vi "measurement.vi"(6 "error in (no error)":errorcluster, 9 "Experiment.lvclass":refnum<class "Experiment.lvclass">) -> (0 "error out":errorcluster, 3 "Experiment out":refnum<class "Experiment.lvclass">)   [LabVIEW 2013, in "Experiment.lvclass"]
doc: "I Description:\nThis example uses a script to manage the generation of a dynamic pattern at a specified clock rate.\n\nII Instructions for Running:\n1. Enter the digital channels on the hardware device to generate digital pattern in the Channel List control.\n2. Specify the clock rate for the generation in the Clock Rate control.\n3. Click the Stop button when you want to stop the generation\n\nIII Block Diagram Steps:\n1. Initialize for a generation session.\n2. Assign specified channels in Channel List for dynamic operation.\n3. Configure the Sample clock to use the onboard clock, and configure the clock rate.\n4. Set the generation mode to Scripted.\n5. Query the Data Width property to determine which Write function to use.\nNote: Different devices have different default values for the Data Width property. If you know the Data Width of your device, you may omit the property node and case structure.\n6. Write digital patterns to the onboard memory of the digital device.\n7. Write the script to the onboard memory.\n8. Initiate dynamic pattern generation.\n9. Wait until the Stop button is clicked or an error occurs, and exit the While loop. \n The niHSDIO Is Done VI is used in the while loop to check only for errors.\n10. Abort generation and close the session.\n\nIV I/O Connections Overview:\nMake connections from output terminals to match the channels specified by Channel List. In this example, the digital pattern is generated from the first 16 digital channels of the device."
uses:
  Experiment.lvclass
  <vilib>/Platform/TimedLoop/XDataNode/timing_clust.ctl
  <vilib>/Platform/TimedLoop/XDataNode/nitl_modes.ctl
  <vilib>/Platform/TimedLoop/XDataNode/wakeup.ctl
  Globals.vi
  <vilib>/platform/TimedLoop/XDataNode/XDataNode.xnode
  <vilib>/Platform/TimedLoop/XDataNode/XDNodeRunTimeDep.lvlib
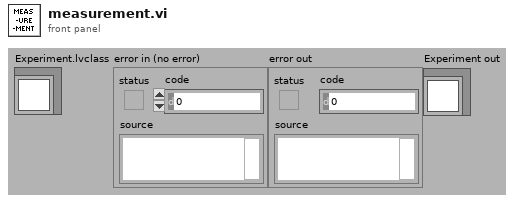
[diagram p1: front panel]
types:
  T1 = typedef "XDNodeRunTimeDep.lvlib/timing_clust.ctl" = cluster{"Expected End [f-1]":u64, "Actual End [f-1]":u64, "Finished Late? [f-1]":bool, "Expected End [i-1]":u64, "Actual End [i-1]":u64, "Finished Late? [i-1]":bool, "Expected Start [i]":u64, "Actual Start [i]":u64, "Expected Start [f]":u64, "Actual Start [f]":u64, "Source Name":string, "Structure Name":string, "Period":i64, "Deadline":i64, "Offset":i64, "Start":i64, "Priority":i32, "Timeout":i32, "Mode":T2, "Wakeup Reason":T3, "Error":errorcluster, "Source Type":string, "Secondary Source Type":string, "Global End Time":u64, "Global Start Time":u64, "Frame Duration":u64, "Iteration Duration":u64, "Assigned CPU":i32, "I/O Scan Engine Mode":u32}
  T2 = typedef "XDNodeRunTimeDep.lvlib/nitl_modes.ctl" = enum32{"No Change", "Process missed periods, maintain original phase", "Discard missed periods, maintain original phase", "Process missed periods, ignore original phase", "Discard missed periods, ignore original phase"}
  T3 = typedef "XDNodeRunTimeDep.lvlib/wakeup.ctl" = enum32{"Normal", "Aborted", "Asynchronous wakeup", "Timing source error", "Timed loop error", "Timeout"}
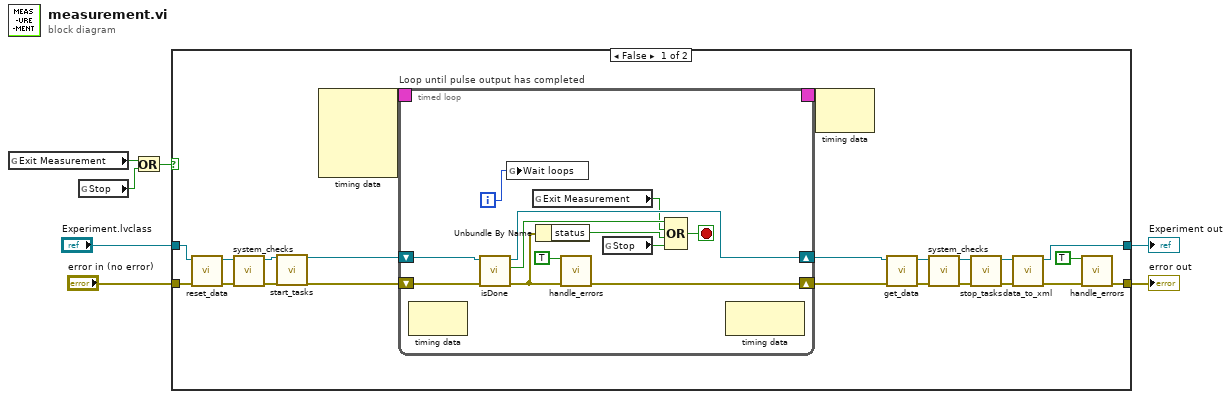
[diagram p0: block diagram]
diagram:
  n1 = global read "Globals.vi" "Exit Measurement"() -> (w3:bool)
  n2 = global read "Globals.vi" "Stop"() -> (w2:bool)
  n3 = Or(x=w3, y=w2) -> (x .or. y?=w1:bool)
  n4 = case shown="False" w1 {
    tunnel: [w13 w46] -> w7
    tunnel: [w12 w47] -> w6
    tunnel: "Experiment.lvclass" -> [w10 w46]
    tunnel: "error in (no error)" -> [w9 w47]
    frame False {
      n5 = call "reset_data.vi"("error in (no error)"=w9, "Experiment in"=w10) -> ("error out"=w19:errorcluster, "Experiment out"=w20:refnum<class "Experiment.lvclass">)  [unwired: 8 in]
      n6 = call "system_checks.vi"("error in (no error)"=w19, "Experiment in"=w20) -> ("error out"=w24:errorcluster, "Experiment out"=w26:refnum<class "Experiment.lvclass">)  [unwired: 8 in]
      n7 = call "start_tasks.vi"("Experiment (in)"=w26, "error in"=w24) -> ("Experiment"=w27:refnum<class "Experiment.lvclass">, "error out"=w25:errorcluster)  [unwired: 16 in]
      n8 = node-c288() -> (w29:T1)  [unwired: 4 in]
      n9 = timed-loop "Loop until pulse output has completed" {
        shift-right: [w30] -> w23
        shift-left: w25 -> [w35]
        timing: w29 -> [_]
        timing-out: [_] -> w28
        shift-right: [w37] -> w22
        shift-left: w27 -> [w38]
        i -> [w36]
        stop <- w41 stop-if-true
        n10 = node-c288() -> ()  [unwired: 1 in, 1 out]
        n11 = call "isDone.vi"("error in (no error)"=w35, "Experiment in"=w38) -> ("error out"=w31:errorcluster, "Is done?"=w39:bool, "Experiment out"=w37:refnum<class "Experiment.lvclass">)  [unwired: 7 in]
        n12 = global write "Globals.vi" "Wait loops"(w36) -> ()
        n13 = global read "Globals.vi" "Exit Measurement"() -> (w34:bool)
        n14 = Unbundle By Name(w31) -> ("status"=w40:bool)
        n15 = call "handle_errors.vi"("Exit Operation"=TRUE ("Exit Measurement"), "error in (no error)"=w31) -> ("error out"=w30:errorcluster)  [unwired: 13 in]
        n16 = global read "Globals.vi" "Stop"() -> (w33:bool)
        n17 = Compound Arithmetic op=OR(w39, w34, w40, w33) -> (w41:bool)
        n18 = node-c288() -> ()  [unwired: 1 in, 1 out]
      }
      n19 = node-c288(w28) -> ()  [unwired: 1 out]
      n20 = call "get_data.vi"("error in (no error)"=w23, "Experiment in"=w22) -> ("error out"=w16:errorcluster, "Experiment out"=w21:refnum<class "Experiment.lvclass">)  [unwired: 8 in]
      n21 = call "system_checks.vi"("error in (no error)"=w16, "Experiment in"=w21) -> ("error out"=w15:errorcluster, "Experiment out"=w18:refnum<class "Experiment.lvclass">)  [unwired: 8 in]
      n22 = call "stop_tasks.vi"("error in (no error)"=w15, "Experiment in"=w18) -> ("error out"=w14:errorcluster, "Experiment out"=w17:refnum<class "Experiment.lvclass">)  [unwired: 8 in]
      n23 = call "data_to_xml.vi"("error in (no error)"=w14, "Experiment in"=w17) -> ("error out"=w8:errorcluster, "Experiment out"=w13:refnum<class "Experiment.lvclass">)  [unwired: 7 in, 1 out]
      n24 = call "handle_errors.vi"("Exit Operation"=TRUE ("Exit Measurement"), "error in (no error)"=w8) -> ("error out"=w12:errorcluster)  [unwired: 13 in]
    }
    frame True {
    }
  }
  "error out" <- w6
  "Experiment out" <- w7
